vi "make_headers.vi"(0 "Method":string="get", 1 "payload":string, 3 "input":T1) -> (7 "signature":string, 10 "output cluster":T1)   [LabVIEW 2019]
uses:
  Downloads/LabVIEW-Bits-master/Cryptographic Services/SHA256/SHA256.lvlib
  <vilib>/Utility/SMTP/NI_SMTPEmail.lvlib
panel:
  out "date from labview":i32
  out "nonce from python":i32
  out "date from python":i32
  out "nonce from labview":i32
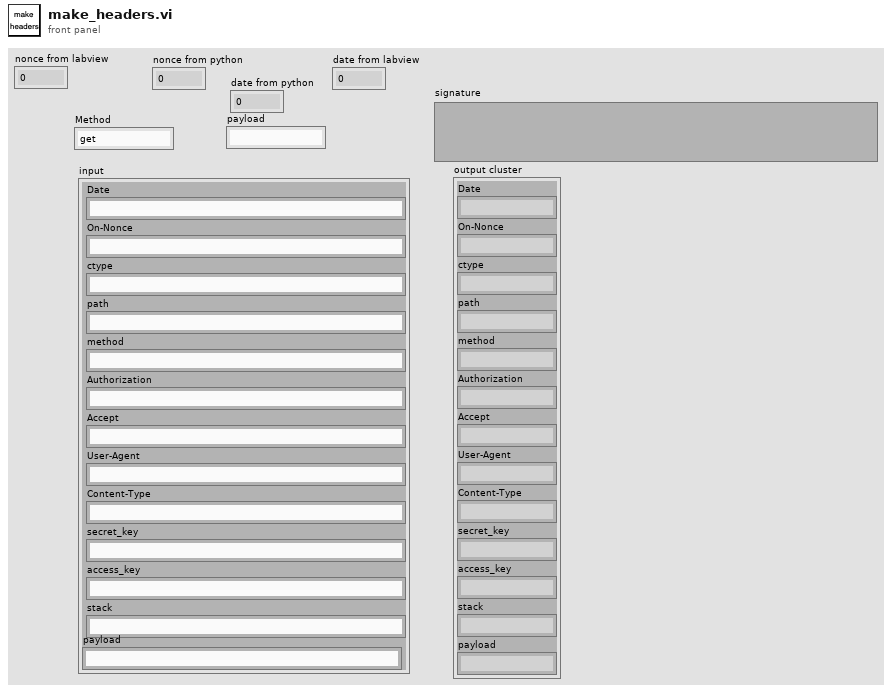
[diagram p1: front panel]
types:
  T1 = cluster{"Date":string, "On-Nonce":string, "ctype":string, "path":string, "method":string, "Authorization":string, "Accept":string, "User-Agent":string, "Content-Type":string, "secret_key":string, "access_key":string, "stack":string, "payload":string}
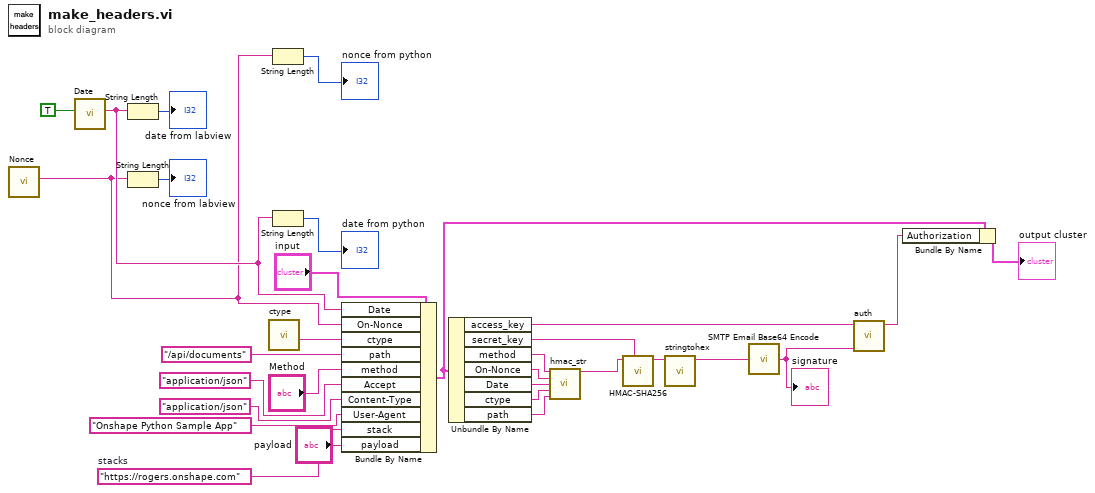
[diagram p0: block diagram]
diagram:
  w11 = "https://rogers.onshape.com"  # stacks
  n1 = call "Nonce.vi"() -> ("delimiter"=w2:string)  [unwired: 11 in]
  n2 = call "Date.vi"("UTC format"=TRUE) -> ("date/time string"=w3:string)  [unwired: 10 in]
  n3 = String Length(string=w3) -> (length=→"date from labview":i32)
  n4 = String Length(string=w2) -> (length=→"nonce from labview":i32)
  n5 = call "ctype.vi"() -> ("ctype"=w29:string)  [unwired: 11 in]
  n6 = String Length(string=w2) -> (length=→"nonce from python":i32)
  n7 = String Length(string=w3) -> (length=→"date from python":i32)
  n8 = Bundle By Name(cluster="input", "Date"=w3, "On-Nonce"=w2, "ctype"=w29, "path"="/api/documents", "method"="Method", "Accept"="application/json" ("Content-Type"), "Content-Type"="application/json" ("Accept"), "User-Agent"="Onshape Python Sample App", "stack"=w11, "payload"="payload") -> (w14:T1)
  n9 = Unbundle By Name(w14) -> ("access_key"=w8:string, "secret_key"=w9:string, "method"=w26:string, "On-Nonce"=w25:string, "Date"=w24:string, "ctype"=w22:string, "path"=w23:string)
  n10 = call "hmac_str.vi"("Method"=w26, "Nonce"=w25, "Date"=w24, "ctype"=w22, "path"=w23) -> ("hmac_str"=w19:string)  [unwired: 9 in, 1 out]
  n11 = call "HMAC-SHA256.vi"("Key"=w9, "String to Encode"=w19) -> ("Hash String"=w21:string)  [unwired: 8 in, 1 out]
  n12 = call "stringtohex.vi"("Hash String"=w21) -> ("string"=w20:string)  [unwired: 10 in]
  n13 = call "SMTP Email Base64 Encode.vi"("Normal String"=w20) -> ("Base64 String"=w15:string)  [unwired: 1 in]
  "signature" <- w15
  n14 = call "auth.vi"("signature"=w15, "access_key"=w8) -> ("auth"=w13:string)  [unwired: 9 in]
  n15 = Bundle By Name(cluster=w14, "Authorization"=w13) -> (→"output cluster":T1)
